vi "GrapRoi.vi"() -> ()   [LabVIEW 2011]
panel:
  in  "ROI Ready":bool
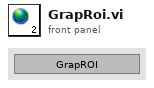
[diagram p1: front panel]
diagram:
